vi "SetupTasks.vi"(9 "eDAQs":T1[][](array[typedef]), 10 "cDAQs":T1[][](array[typedef]), 11 "PXI":T1[][](array[typedef])) -> (0 "cDAQ i":i32[](array[numeric]), 1 "eDAQ i":i32[][](array[numeric]), 2 "cDAQs":refnum<k21>[](array[refnum]), 3 "eDAQs":refnum<k21>[](array[refnum]), 4 "PXI i":i32[][](array[numeric]), 5 "PXIs":refnum<k21>[](array[refnum]))   [LabVIEW 2013]
uses:
  Channels_and_Index.ctl
  Globals/Meas_global.vi
  <vilib>/DAQmx/create/channels.llb/DAQmx Create Channel (AI-Voltage-Basic).vi
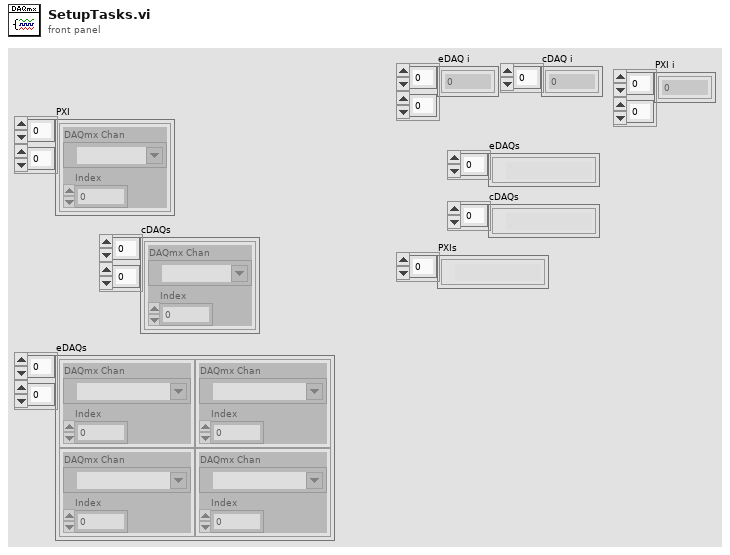
[diagram p1: front panel]
types:
  T1 = typedef "Channels_and_Index.ctl" = cluster{"DAQmx Chan":tag, "Index":i32}
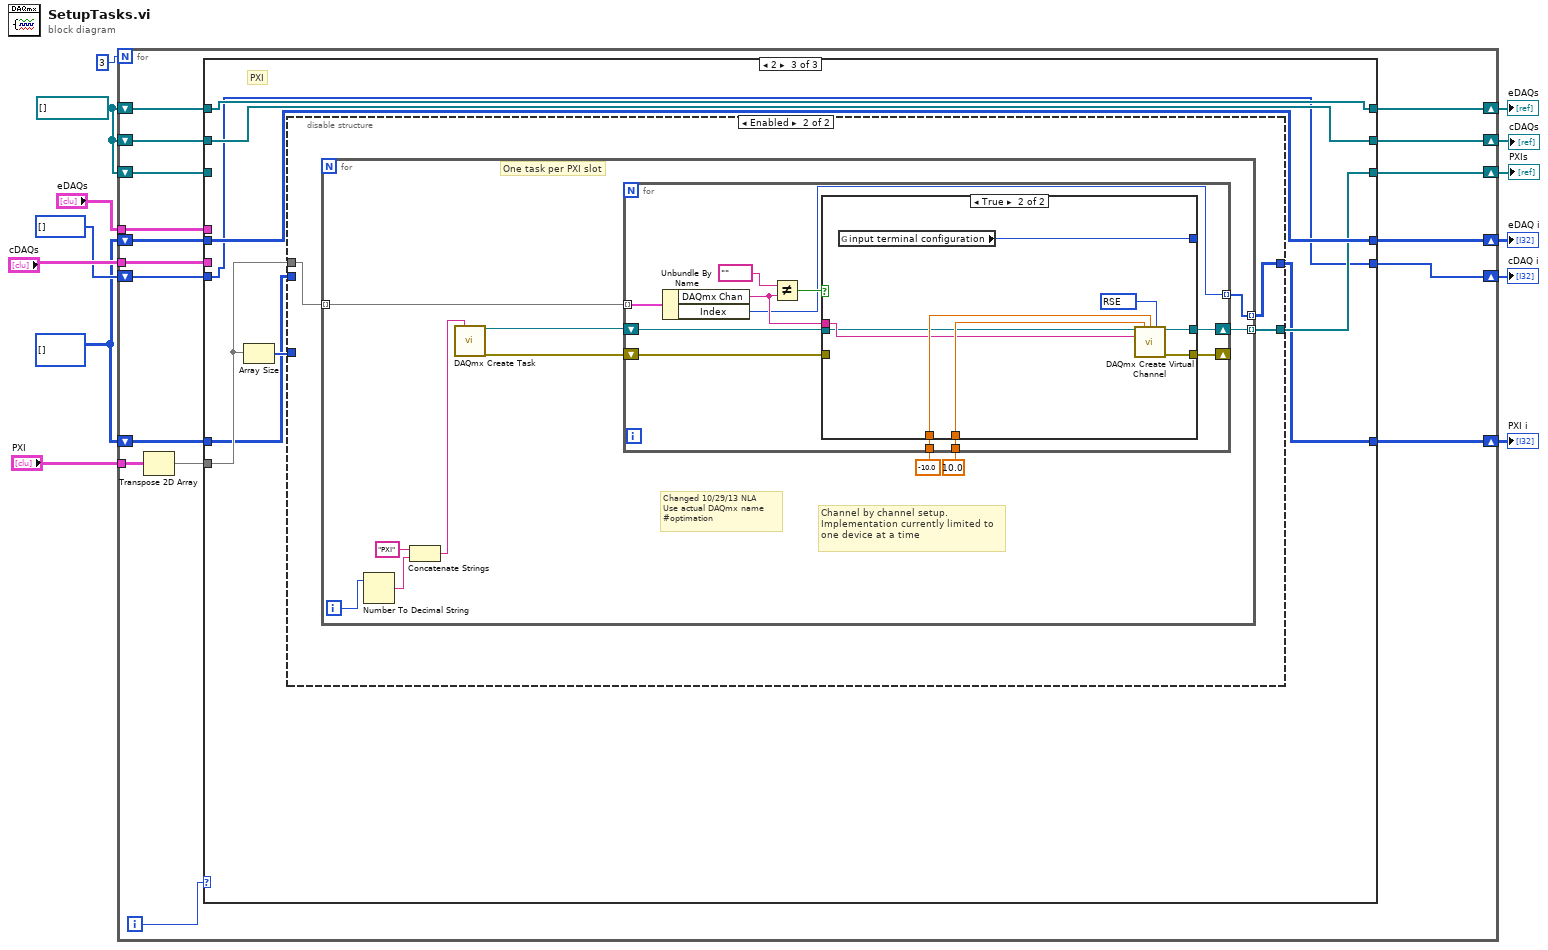
[diagram p0: block diagram]
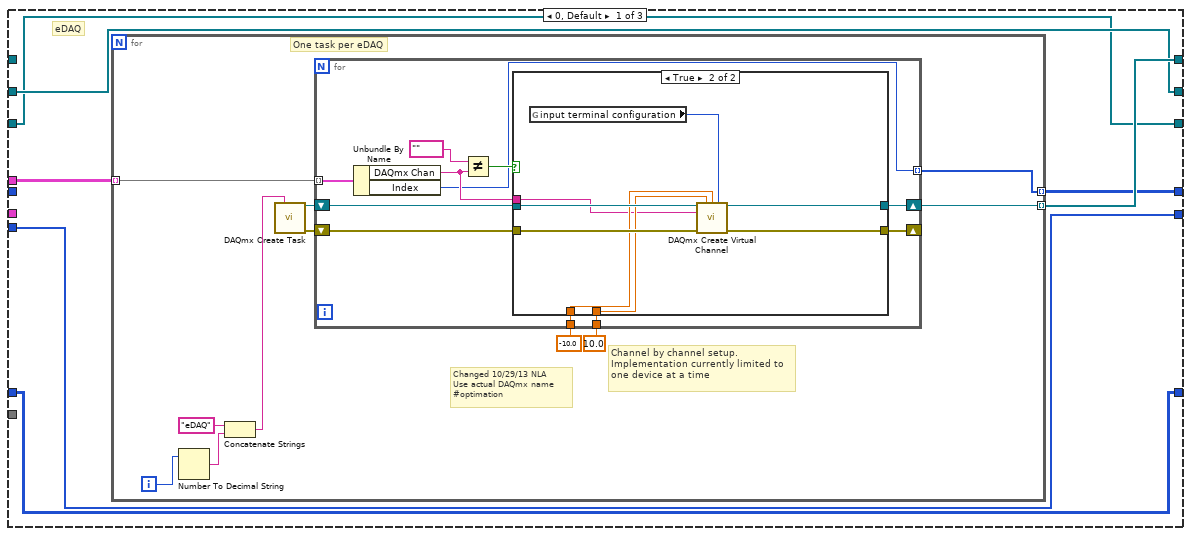
[diagram p2: hidden frame]
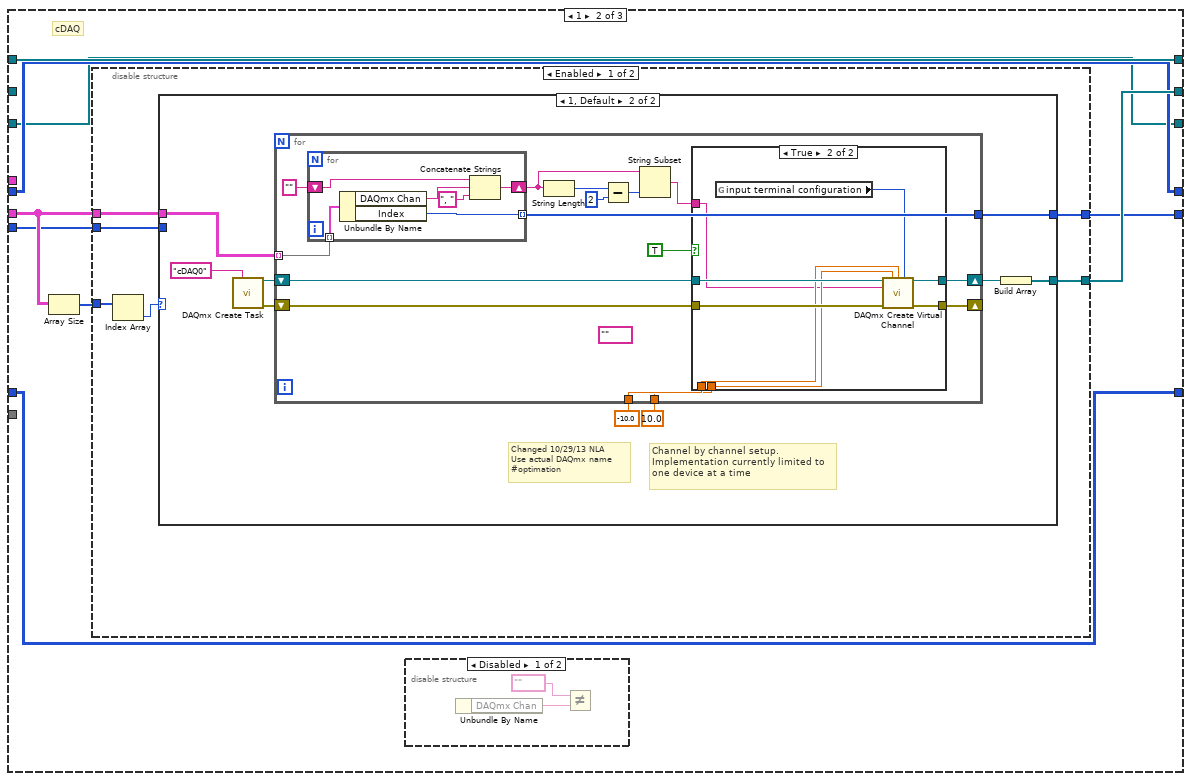
[diagram p4: hidden frame]
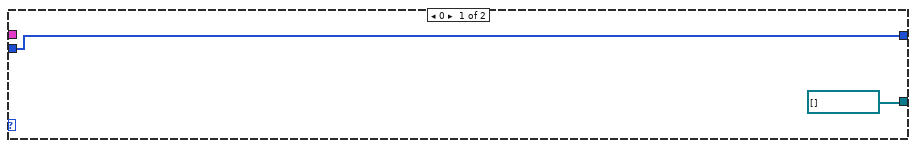
[diagram p6: hidden frame]
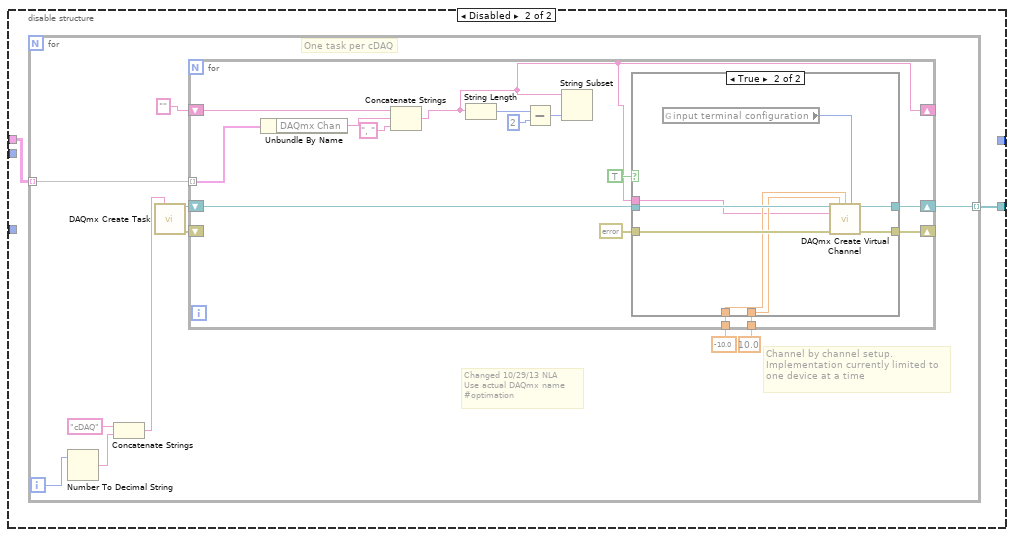
[diagram p8: hidden frame]
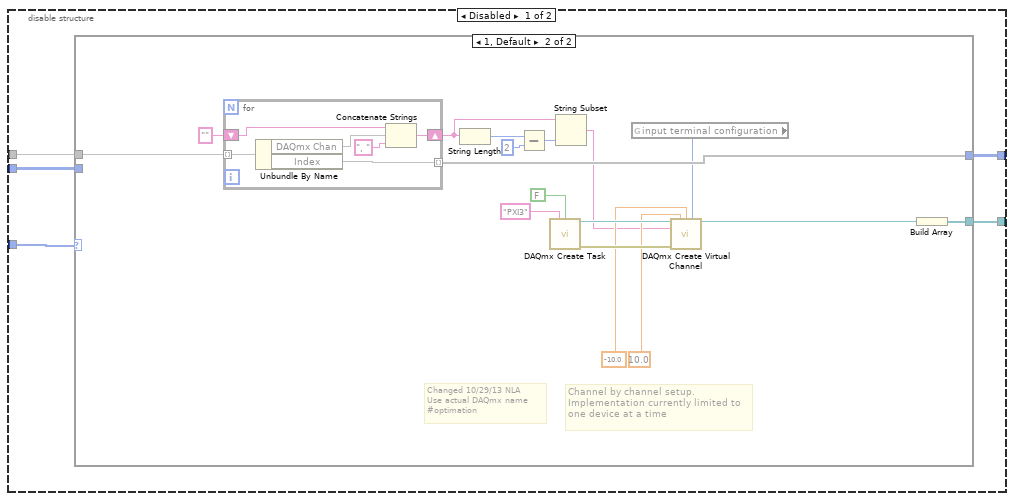
[diagram p10: hidden frame]
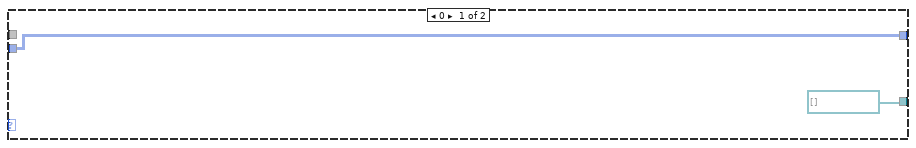
[diagram p11: hidden frame]
diagram:
  w1 = i32[][] []
  w6 = refnum<k21>[] []
  n1 = for {
    N: 3 -> [_]
    tunnel: "eDAQs" -> [w30]
    shift-right: [w29] -> w11
    shift-left: w6 -> [w27]
    tunnel: "cDAQs" -> [w26]
    shift-right: [w25] -> w10
    shift-left: w6 -> [w24]
    shift-right: [w23] -> w7
    shift-left: w1 -> [w22]
    shift-right: [w21] -> w8
    shift-left: i32[] [] -> [w20]
    shift-right: [w16] -> w5
    shift-left: w6 -> [w19]
    shift-right: [w15] -> w2
    shift-left: w1 -> [w18]
    tunnel: "PXI" -> [w17]
    i -> [w28]
    n2 = Transpose 2D Array(2D array=w17) -> (transposed array=w14:T1[][])
    n3 = case shown="2" w28 {
      tunnel: w30 -> [w37 _ _]
      tunnel: [w36 w78 w175] -> w29
      tunnel: w27 -> [_ w78 w175]
      tunnel: w26 -> [_ w77 _]
      tunnel: [w35 w75 w171] -> w25
      tunnel: w24 -> [w35 _ w171]
      tunnel: [w34 w74 w173] -> w23
      tunnel: w22 -> [_ w74 w173]
      tunnel: [w33 w73 w169] -> w21
      tunnel: w20 -> [w33 w72 w169]
      tunnel: w19 -> [w32 w71 _]
      tunnel: w18 -> [w31 w70 w168]
      tunnel: w14 -> [_ _ w172]
      tunnel: [w32 w71 w170] -> w16
      tunnel: [w31 w70 w167] -> w15
      frame 0, Default {
        # "eDAQ"
        n4 = for {
          tunnel: w37 -> [w44] mode=indexing
          tunnel: [w43] -> w36 mode=indexing
          tunnel: [w38] -> w34 mode=indexing
          i -> [w42]
          # "One task per eDAQ"
          # "Changed 10/29/13 NLA\nUse actual DAQmx name\n#optimation"
          # "Channel by channel setup. Implementation currently limited to one device at a time"
          n5 = Number To Decimal String(number=w42) -> (decimal integer string=w41:string)  [unwired: 1 in]
          n6 = Concatenate Strings("eDAQ" ("string"), w41) -> (w39:string)
          n7 = call <vilib>:"DAQmx Create Task.vi"("new task name"=w39) -> ("task out"=w47:refnum<k21>, "error out"=w48:errorcluster)  [unwired: 4 in, 9 out]
          n8 = for {
            shift-right: [w58] -> w43
            shift-left: w47 -> [w59]
            shift-right: [w56] -> _
            shift-left: w48 -> [w57]
            tunnel: -10.0 -> [w55]
            tunnel: 10.0 -> [w54]
            tunnel: w44 -> [w53] mode=indexing
            tunnel: [w49] -> w38 mode=indexing
            n9 = Unbundle By Name(w53) -> ("DAQmx Chan"=w50:tag, "Index"=w49:i32)
            n10 = Not Equal?(x=tag "", y=w50) -> (x != y?=w51:bool)
            n11 = case shown="True" w51 {
              tunnel: w59 -> [w61 w69]
              tunnel: [w61 w68] -> w58
              tunnel: w57 -> [w60 w67]
              tunnel: [w60 w66] -> w56
              tunnel: w55 -> [_ w65]
              tunnel: w54 -> [_ w64]
              tunnel: w50 -> [_ w62]
              frame False {
              }
              frame True {
                n12 = global read "Meas_global.vi" "input terminal configuration"() -> (w63:i32)
                n13 = call-poly <vilib>:"DAQmx Create Virtual Channel.vi"("task in"=w69, "maximum value"=w64, "minimum value"=w65, "input terminal configuration"=w63, "physical channels"=w62, "error in"=w67) -> ("task out"=w68:refnum<k21>, "error out"=w66:errorcluster)  [unwired: 3 in, 5 out]
              }
            }
          }
        }
      }
      frame 1 {
        # "cDAQ"
        n14 = Array Size(array=w77) -> (size(s)=w76:i32[])
        n15 = disable-structure shown="Enabled" {
          disable-tunnel: w77 -> [w86 w129]
          disable-tunnel: w76 -> [w85 _]
          disable-tunnel: [w84 w130] -> w75
          disable-tunnel: [w82 _] -> w73
          disable-tunnel: w72 -> [w81 _]
          frame Enabled {
            n16 = Index Array(array=w85) -> (element=w83:i32)  [unwired: 1 in]
            n17 = case shown="1, Default" w83 {
              tunnel: w86 -> [_ w97]
              tunnel: [refnum<k21>[] [] w90] -> w84
              tunnel: [w87 w89] -> w82
              tunnel: w81 -> [w87 _]
              frame 0 {
              }
              frame 1, Default {
                # "Changed 10/29/13 NLA\nUse actual DAQmx name\n#optimation"
                # "Channel by channel setup. Implementation currently limited to one device at a time"
                n18 = call <vilib>:"DAQmx Create Task.vi"("new task name"="cDAQ0") -> ("task out"=w95:refnum<k21>, "error out"=w96:errorcluster)  [unwired: 4 in, 9 out]
                n19 = for {
                  shift-right: [w112] -> w92
                  shift-left: w95 -> [w99]
                  shift-right: [w110] -> _
                  shift-left: w96 -> [w111]
                  tunnel: -10.0 -> [w109]
                  tunnel: 10.0 -> [w108]
                  tunnel: w97 -> [w102] mode=indexing
                  tunnel: [w98] -> w89
                  (unwired) tag "" ("x")
                  n20 = for {
                    shift-right: [w116] -> w104
                    shift-left: "" -> [w115]
                    tunnel: w102 -> [w114] mode=indexing
                    tunnel: [w113] -> w98 mode=indexing
                    n21 = Unbundle By Name(w114) -> ("DAQmx Chan"=w118:tag, "Index"=w113:i32)
                    n22 = Concatenate Strings(w115, w118, ", " ("string")) -> (w116:string)
                  }
                  n23 = String Length(string=w104) -> (length=w106:i32)
                  n24 = Subtract(x=w106, y=2) -> (x-y=w105:i32)
                  n25 = String Subset(string=w104, length (rest)=w105) -> (substring=w101:string)  [unwired: 1 in]
                  n26 = case shown="True" TRUE {
                    tunnel: w99 -> [w120 w128]
                    tunnel: [w120 w127] -> w112
                    tunnel: w111 -> [w119 w126]
                    tunnel: [w119 w125] -> w110
                    tunnel: w109 -> [_ w124]
                    tunnel: w108 -> [_ w123]
                    tunnel: w101 -> [_ w121]
                    frame False {
                    }
                    frame True {
                      n27 = global read "Meas_global.vi" "input terminal configuration"() -> (w122:i32)
                      n28 = call-poly <vilib>:"DAQmx Create Virtual Channel.vi"("task in"=w128, "maximum value"=w123, "minimum value"=w124, "input terminal configuration"=w122, "physical channels"=w121, "error in"=w126) -> ("task out"=w127:refnum<k21>, "error out"=w125:errorcluster)  [unwired: 3 in, 5 out]
                    }
                  }
                }
                n29 = Build Array(w92) -> (w90:refnum<k21>[])
              }
            }
          }
          frame Disabled {
            n30 = for {
              tunnel: w129 -> [w137] mode=indexing
              tunnel: [w136] -> w130 mode=indexing
              i -> [w135]
              # "One task per cDAQ"
              # "Changed 10/29/13 NLA\nUse actual DAQmx name\n#optimation"
              # "Channel by channel setup. Implementation currently limited to one device at a time"
              n31 = Number To Decimal String(number=w135) -> (decimal integer string=w134:string)  [unwired: 1 in]
              n32 = Concatenate Strings("cDAQ" ("string"), w134) -> (w132:string)
              n33 = call <vilib>:"DAQmx Create Task.vi"("new task name"=w132) -> ("task out"=w140:refnum<k21>, "error out"=w141:errorcluster)  [unwired: 4 in, 9 out]
              n34 = for {
                shift-right: [w155] -> w136
                shift-left: w140 -> [w156]
                shift-right: [w154] -> _
                shift-left: w141 -> [_]
                tunnel: -10.0 -> [w153]
                tunnel: 10.0 -> [w152]
                tunnel: w137 -> [w148] mode=indexing
                shift-right: [w143] -> _
                shift-left: "" -> [w144]
                n35 = Unbundle By Name(w148) -> ("DAQmx Chan"=w146:tag)
                n36 = Concatenate Strings(w144, w146, ", " ("string")) -> (w143:string)
                n37 = String Length(string=w143) -> (length=w150:i32)
                n38 = Subtract(x=w150, y=2) -> (x-y=w151:i32)
                n39 = String Subset(string=w143, length (rest)=w151) -> ()  [unwired: 1 in, 1 out]
                n40 = case shown="True" TRUE {
                  tunnel: w156 -> [w158 w166]
                  tunnel: [w158 w165] -> w155
                  tunnel: errorcluster {"status"=FALSE, "code"=0, "source"=""} ("error out") -> [w157 w164]
                  tunnel: [w157 w159] -> w154
                  tunnel: w153 -> [_ w163]
                  tunnel: w152 -> [_ w162]
                  tunnel: w143 -> [_ w160]
                  frame False {
                  }
                  frame True {
                    n41 = global read "Meas_global.vi" "input terminal configuration"() -> (w161:i32)
                    n42 = call-poly <vilib>:"DAQmx Create Virtual Channel.vi"("task in"=w166, "maximum value"=w162, "minimum value"=w163, "input terminal configuration"=w161, "physical channels"=w160, "error in"=w164) -> ("task out"=w165:refnum<k21>, "error out"=w159:errorcluster)  [unwired: 3 in, 5 out]
                  }
                }
              }
            }
          }
        }
        n43 = disable-structure shown="Disabled" {
          frame Disabled {
            n44 = Unbundle By Name() -> ("DAQmx Chan"=w80:tag)  [unwired: 1 in]
            n45 = Not Equal?(x=tag "", y=w80) -> ()  [unwired: 1 out]
          }
          frame Enabled {
          }
        }
      }
      frame 2 {
        # "PXI"
        n46 = Array Size(array=w172) -> (size(s)=w174:i32[])
        n47 = disable-structure shown="Enabled" {
          disable-tunnel: w172 -> [w180 w208]
          disable-tunnel: w174 -> [w176 _]
          disable-tunnel: [w179 w206] -> w170
          disable-tunnel: [w178 w207] -> w167
          disable-tunnel: w168 -> [w177 _]
          frame Disabled {
            n48 = case shown="1, Default" w176 {
              tunnel: w180 -> [_ w199]
              tunnel: [refnum<k21>[] [] w192] -> w179
              tunnel: [w181 w191] -> w178
              tunnel: w177 -> [w181 _]
              frame 0 {
              }
              frame 1, Default {
                # "Changed 10/29/13 NLA\nUse actual DAQmx name\n#optimation"
                # "Channel by channel setup. Implementation currently limited to one device at a time"
                n49 = for {
                  shift-right: [w203] -> w187
                  shift-left: "" -> [w202]
                  tunnel: w199 -> [w201] mode=indexing
                  tunnel: [w200] -> w191 mode=indexing
                  n50 = Unbundle By Name(w201) -> ("DAQmx Chan"=w205, "Index"=w200)
                  n51 = Concatenate Strings(w202, w205, ", " ("string")) -> (w203:string)
                }
                n52 = String Length(string=w187) -> (length=w189:i32)
                n53 = Subtract(x=w189, y=2) -> (x-y=w188:i32)
                n54 = call <vilib>:"DAQmx Create Task.vi"("new task name"="PXI3", "auto cleanup"=FALSE) -> ("task out"=w197:refnum<k21>, "error out"=w198:errorcluster)  [unwired: 3 in, 9 out]
                n55 = String Subset(string=w187, length (rest)=w188) -> (substring=w185:string)  [unwired: 1 in]
                n56 = global read "Meas_global.vi" "input terminal configuration"() -> (w184:i32)
                n57 = call-poly <vilib>:"DAQmx Create Virtual Channel.vi"("task in"=w197, "maximum value"=10.0, "minimum value"=-10.0, "input terminal configuration"=w184, "physical channels"=w185, "error in"=w198) -> ("task out"=w194:refnum<k21>)  [unwired: 3 in, 6 out]
                n58 = Build Array(w194) -> (w192:refnum<k21>[])
              }
            }
          }
          frame Enabled {
            n59 = for {
              tunnel: w208 -> [w217] mode=indexing
              tunnel: [w216] -> w206 mode=indexing
              tunnel: [w211] -> w207 mode=indexing
              i -> [w215]
              # "One task per PXI slot"
              # "Changed 10/29/13 NLA\nUse actual DAQmx name\n#optimation"
              # "Channel by channel setup. Implementation currently limited to one device at a time"
              n60 = Number To Decimal String(number=w215) -> (decimal integer string=w214:string)  [unwired: 1 in]
              n61 = Concatenate Strings("PXI" ("string"), w214) -> (w212:string)
              n62 = call <vilib>:"DAQmx Create Task.vi"("new task name"=w212) -> ("task out"=w210:refnum<k21>, "error out"=w209:errorcluster)  [unwired: 4 in, 9 out]
              n63 = for {
                shift-right: [w229] -> w216
                shift-left: w210 -> [w230]
                shift-right: [w227] -> _
                shift-left: w209 -> [w228]
                tunnel: -10.0 -> [w226]
                tunnel: 10.0 -> [w225]
                tunnel: w217 -> [w224] mode=indexing
                tunnel: [w220] -> w211 mode=indexing
                n64 = Unbundle By Name(w224) -> ("DAQmx Chan"=w221:tag, "Index"=w220:i32)
                n65 = Not Equal?(x=tag "", y=w221) -> (x != y?=w222:bool)
                n66 = case shown="True" w222 {
                  tunnel: w230 -> [w232 w235]
                  tunnel: [w232 w240] -> w229
                  tunnel: w228 -> [w231 _]
                  tunnel: [w231 w239] -> w227
                  tunnel: w226 -> [_ w238]
                  tunnel: w225 -> [_ w237]
                  tunnel: w221 -> [_ w236]
                  tunnel: [_ w233] -> _
                  frame False {
                  }
                  frame True {
                    w234 = 10083 items=["default"=-1, "RSE"=10083, "NRSE"=10078, "Differential"=10106, "Pseudodifferential"=12529] ("input terminal configuration")
                    n67 = global read "Meas_global.vi" "input terminal configuration"() -> (w233:i32)
                    n68 = call-poly <vilib>:"DAQmx Create Virtual Channel.vi"("task in"=w235, "maximum value"=w237, "minimum value"=w238, "input terminal configuration"=w234, "physical channels"=w236) -> ("task out"=w240:refnum<k21>, "error out"=w239:errorcluster)  [unwired: 4 in, 5 out]
                  }
                }
              }
            }
          }
        }
      }
    }
  }
  "eDAQs" <- w11
  "cDAQs" <- w10
  "cDAQ i" <- w8
  "eDAQ i" <- w7
  "PXIs" <- w5
  "PXI i" <- w2
